vi "Get Tx Configuration.vi"(8 "error in":errorcluster, 10 "configuration string":string, 11 "custom device":T1 format="%.0x") -> (0 "error out":errorcluster, 2 "configuration string out":string, 3 "custom device out":T1 format="%.0x")   [LabVIEW 2020, in "Ballard ARINC 429 Hardware Configuration.lvlib"]
uses:
  Ballard ARINC 429 Hardware Configuration.lvlib
  <vilib>/NI VeriStand/Custom Device API/Custom Device Item Ref.ctl
  Scripting/Ballard/Ballard ARINC 429 Scripting.lvlib
  Scripting/ARINC 429/ARINC 429 Scripting.lvlib
  <vilib>/NI VeriStand/Custom Device API/Custom Device API.lvlib
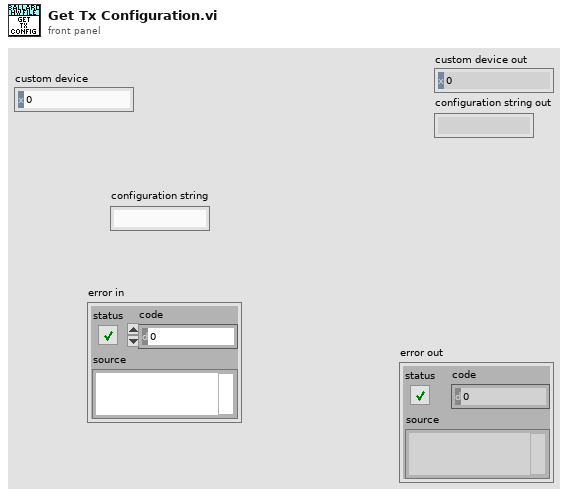
[diagram p1: front panel]
types:
  T1 = typedef "Custom Device API.lvlib/Custom Device Item Ref.ctl" = u64
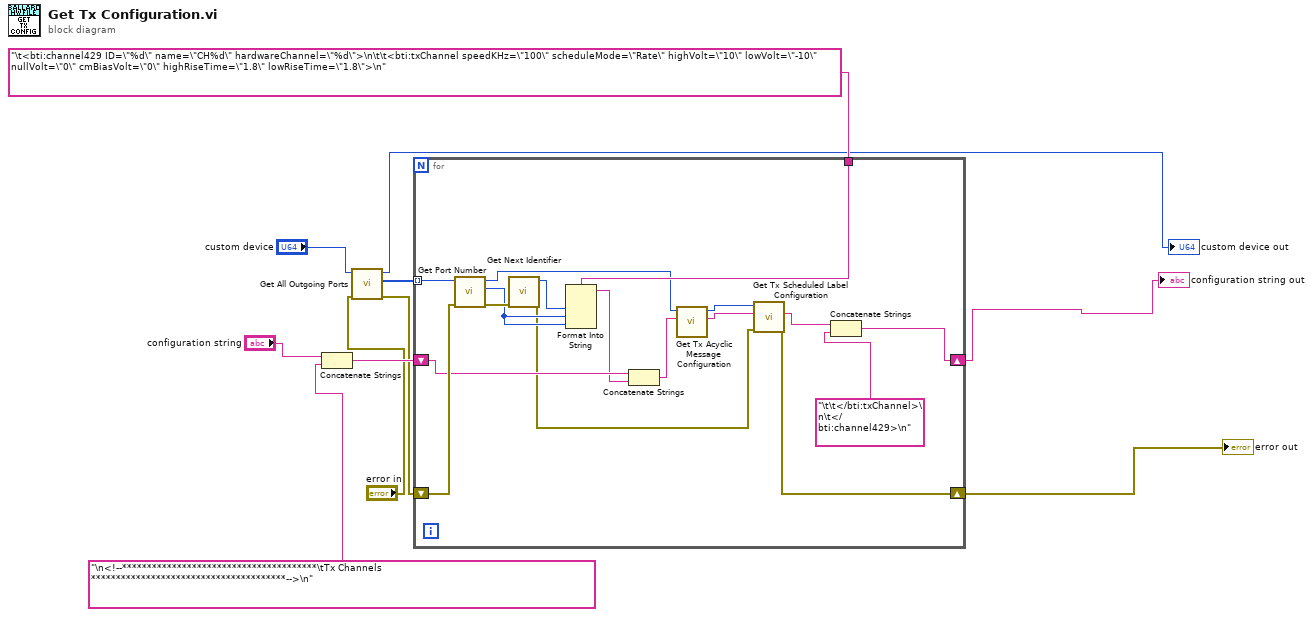
[diagram p0: block diagram]
diagram:
  n1 = Concatenate Strings("configuration string", "\n<!--***************************************\tTx Channels ***************************************-->\n") -> (w7:string)
  n2 = call "Get All Outgoing Ports.vi"("error in"="error in", "Ballard ARINC 429 custom device in"="custom device") -> ("error out"=w2:errorcluster, "outgoing ports"=w8:T1[], "Ballard ARINC 429 custom device out"=→"custom device out":T1)  [unwired: 7 in]
  n3 = for {
    tunnel: w8 -> [w28] mode=indexing
    shift-right: [w16] -> w1
    shift-left: w7 -> [w23]
    shift-right: [w19] -> w5
    shift-left: w2 -> [w27]
    tunnel: "\t<bti:channel429 ID=\"%d\" name=\"CH%d\" hardwareChannel=\"%d\">\n\t\t<bti:txChannel speedKHz=\"100\" scheduleMode=\"Rate\" highVolt=\"10\" lowVolt=\"-10\" nullVolt=\"0\" cmBiasVolt=\"0\" highRiseTime=\"1.8\" lowRiseTime=\"1.8\">\n" -> [w25]
    n4 = call "Get Port Number.vi"("error in"=w27, "port ref in"=w28) -> ("error out"=w26:errorcluster, "port number"=w21:u16, "port ref out"=w14:T1)  [unwired: 6 in, 1 out]
    n5 = call "Get Next Identifier.vi"("error in"=w26) -> ("error out"=w20:errorcluster, "ID"=w24:u32)  [unwired: 9 in]
    n6 = Format Into String(format string=w25, w24, w21, w21) -> (resulting string=w22:string)  [unwired: 2 in, 1 out]
    n7 = Concatenate Strings(w23, w22) -> (w15:string)
    n8 = call "Get Tx Acyclic Message Configuration.vi"("configuration string"=w15, "port"=w14) -> ("configuration string out"=w13:string, "port out"=w12:T1)  [unwired: 7 in, 1 out]
    n9 = call "Get Tx Scheduled Label Configuration.vi"("error in"=w20, "configuration string"=w13, "port"=w12) -> ("error out"=w19:errorcluster, "configuration string out"=w18:string)  [unwired: 6 in, 1 out]
    n10 = Concatenate Strings(w18, "\t\t</bti:txChannel>\n\t</bti:channel429>\n") -> (w16:string)
  }
  "error out" <- w5
  "configuration string out" <- w1
